vi "write_attributes.vi"(8 "error in (no error)":errorcluster, 10 "attributes":T1, 11 "MultiTaskElasticNetCV in":refnum<class "MultiTaskElasticNetCV.lvclass">) -> (0 "error out":errorcluster, 3 "MultiTaskElasticNetCV out":refnum<class "MultiTaskElasticNetCV.lvclass">)   [LabVIEW 2020, in "MultiTaskElasticNetCV.lvclass"]
uses:
  MultiTaskElasticNetCV.lvclass
  Controls/multi_task_elasticnet_cv_attributes.ctl
  MultiTaskElasticNetCV.lvclass/MultiTaskElasticNetCV.ctl
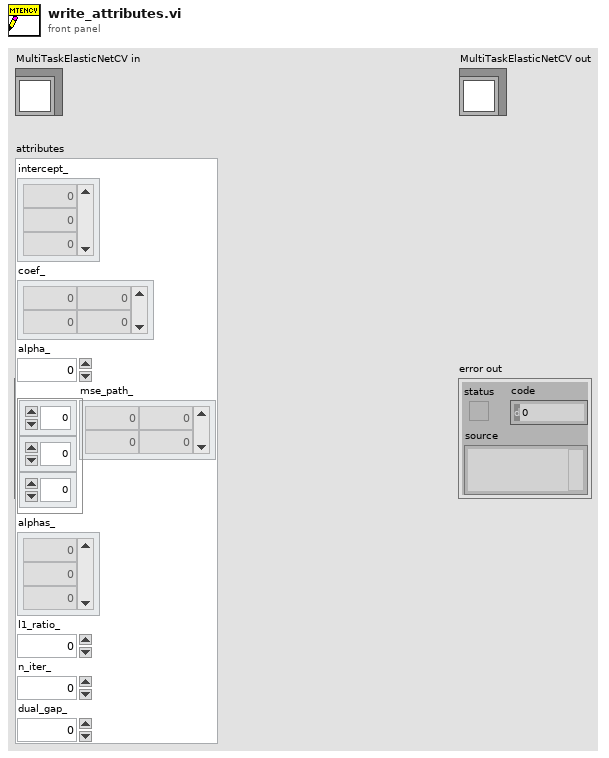
[diagram p1: front panel]
types:
  T1 = typedef "multi_task_elasticnet_cv_attributes.ctl" = cluster{"intercept_":dbl[], "coef_":dbl[][], "alpha_":dbl, "mse_path_":dbl[][][], "alphas_":dbl[], "l1_ratio_":dbl, "n_iter_":dbl, "dual_gap_":dbl}
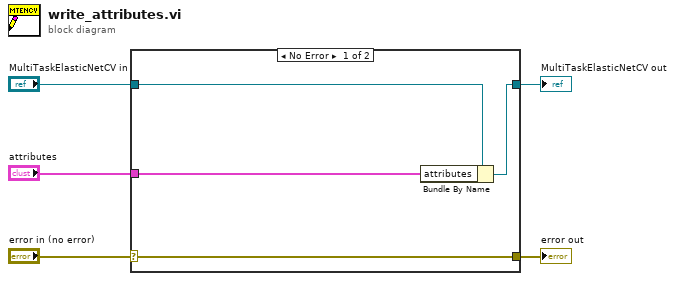
[diagram p0: block diagram]
diagram:
  n1 = case shown="No Error" "error in (no error)" {
    selector: "error in (no error)" -> [w9 w10]
    tunnel: [w9 w10] -> w4
    tunnel: [w7 w11] -> w2
    tunnel: "MultiTaskElasticNetCV in" -> [w8 w11]
    tunnel: "attributes" -> [w6 _]
    frame No Error {
      n2 = Bundle By Name(cluster=w8, "attributes"=w6) -> (w7:refnum<class "MultiTaskElasticNetCV.lvclass">)
    }
    frame Error {
    }
  }
  "error out" <- w4
  "MultiTaskElasticNetCV out" <- w2
